vi "Modify VI Settings.vi"() -> ()   [LabVIEW 2013]
uses:
  ReentrancyType--Enum.ctl
panel:
  in  "Set Reentrancy Type":bool=TRUE
  in  "Set Inline":bool=TRUE
  in  "Set Auto Error Handling":bool=TRUE
  in  "Set Debugging":bool=TRUE
  in  "Path":path=path "C:/Project/JKI-Internal/OpenG-Variant-Data-Library/source"
  in  "Exceptions (VI Names)":string[](array[string])=["Size of Data from TD", "Get Default Data from TD"]
  in  "Reentrancy Type":T1=enum."Preallocate Reentrant"
  in  "Inline":bool=TRUE
  in  "Automatic Error Handling":bool
  in  "Debugging":bool
  # "Settings"
  # "Set?"
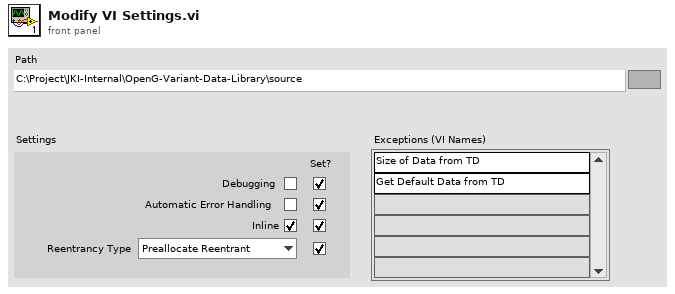
[diagram p1: front panel]
types:
  T1 = typedef "ReentrancyType--Enum.ctl" = enum16{"Non Reentrant", "Shared Clones Reentrant", "Preallocate Reentrant"}
  T2 = enum32{"invalid VI type", "Standard VI", "Control VI", "Global VI", "Polymorphic VI", "Configuration VI", "SubSystem", "Facade VI", "Method VI", "Statechart Diagram VI"}
  T3 = enum16{"Share clones between instances", "Preallocate clone for each instance"}
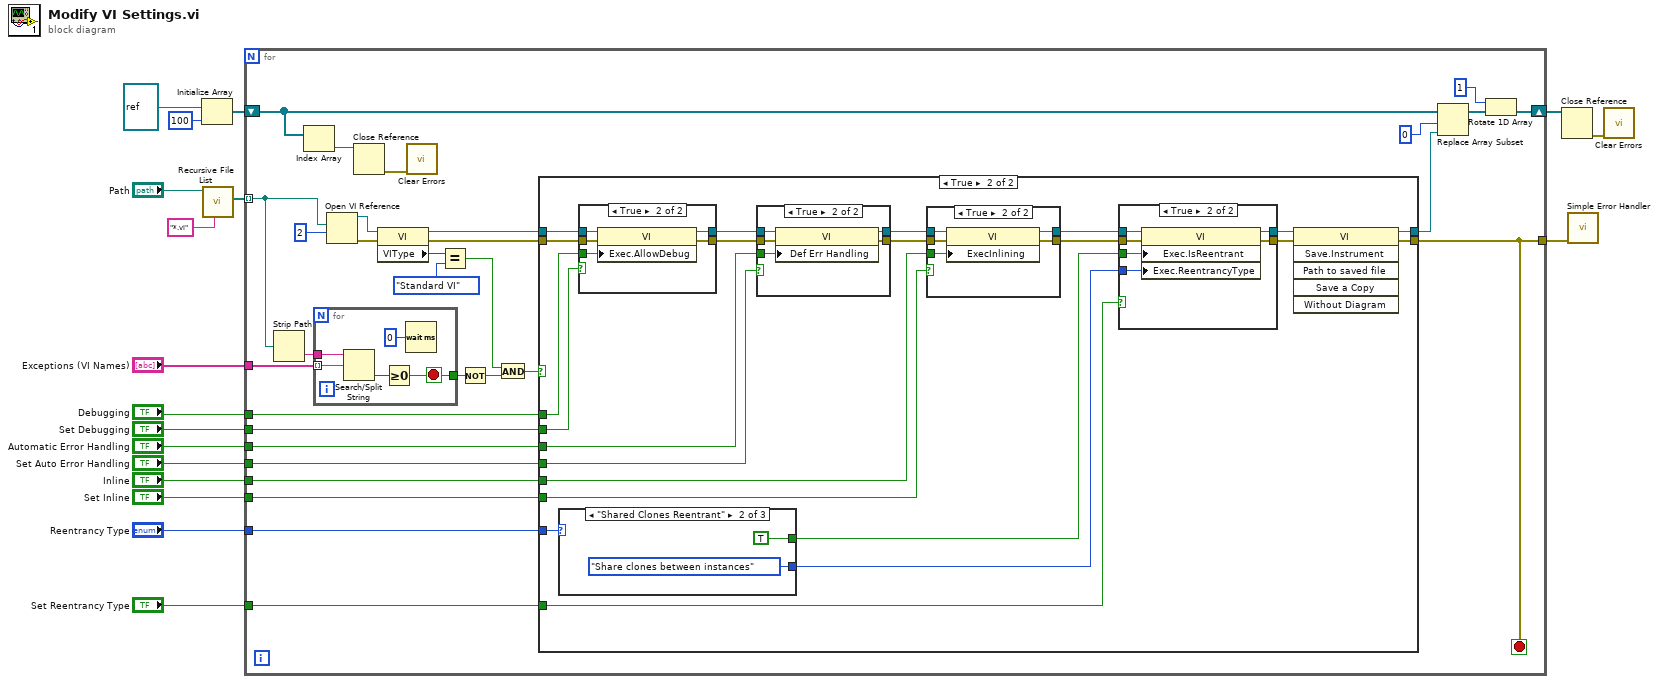
[diagram p0: block diagram]
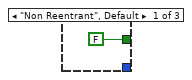
[diagram p7: hidden frame]
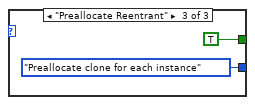
[diagram p8: hidden frame]
diagram:
  n1 = Initialize Array(refnum<vi> refnum ("vi reference"), 100 ("dimension size")) -> (w15:refnum<vi>[])
  n2 = call <vilib>:"Recursive File List.vi"("pattern"="*.vi", "Folder Path"="Path") -> ("All Files in Dir"=w13:path[])  [unwired: 5 in, 4 out]
  n3 = for {
    tunnel: w13 -> [w46] mode=indexing
    tunnel: "Debugging" -> [w48]
    tunnel: "Automatic Error Handling" -> [w47]
    tunnel: "Exceptions (VI Names)" -> [w45]
    shift-right: [w41] -> w7
    shift-left: w15 -> [w39]
    tunnel: [w30] -> w14
    tunnel: "Reentrancy Type" -> [w32]
    tunnel: "Inline" -> [w31]
    tunnel: "Set Debugging" -> [w22]
    tunnel: "Set Auto Error Handling" -> [w21]
    tunnel: "Set Inline" -> [w20]
    tunnel: "Set Reentrancy Type" -> [w19]
    stop <- w30 stop-if-true
    n4 = Strip Path(path=w46) -> (name=w44:string)  [unwired: 1 out]
    n5 = Index Array(array=w39) -> (element=w38:refnum<vi>)  [unwired: 1 in]
    n6 = for {
      tunnel: w45 -> [w110] mode=indexing
      tunnel: w44 -> [w111]
      tunnel: [w108] -> w26
      stop <- w108 stop-if-true
      n7 = Search/Split String(string=w111, search string/char (-)=w110) -> (offset of match=w112:i32)  [unwired: 1 in, 2 out]
      n8 = Greater Or Equal To 0?(x=w112) -> (x >= 0?=w108:bool)
      n9 = Wait (ms)(milliseconds to wait=u32 0) -> ()  [unwired: 1 out]
    }
    n10 = Open VI Reference(vi path=w46, options=2) -> (vi reference=w34:refnum<vi>, error out=w49:errorcluster)  [unwired: 4 in]
    n11 = Close Reference(reference=w38) -> (error out=w37:errorcluster)  [unwired: 1 in]
    n12 = property class="VI"(reference=w34, error in=w49) -> (reference out=w33:refnum<vi>, error out=w35:errorcluster, "VIType"=w28:T2)
    n13 = call <vilib>:"Clear Errors.vi"("error in (no error)"=w37) -> ()  [unwired: 6 in, 1 out]
    n14 = Equal?(x=w28, y=T2."Standard VI") -> (x = y?=w27:bool)
    n15 = Not(x=w26) -> (.not. x?=w25:bool)
    n16 = And(x=w27, y=w25) -> (x .and. y?=w24:bool)
    n17 = case shown="True" w24 {
      tunnel: w48 -> [_ w64]
      tunnel: w47 -> [_ w60]
      tunnel: [w50 w71] -> w29
      tunnel: [w51 w70] -> w30
      tunnel: w35 -> [w51 w65]
      tunnel: w33 -> [w50 w66]
      tunnel: w32 -> [_ w67]
      tunnel: w31 -> [_ w55]
      tunnel: w22 -> [_ w63]
      tunnel: w21 -> [_ w59]
      tunnel: w20 -> [_ w54]
      tunnel: w19 -> [_ w52]
      frame False {
      }
      frame True {
        n18 = case shown="\"Shared Clones Reentrant\"" w67 {
          tunnel: [_ T3."Share clones between instances" ("Execution:Reentrancy Type") T3."Preallocate clone for each instance" ("Execution:Reentrancy Type")] -> w69
          tunnel: [FALSE TRUE TRUE] -> w68
          frame "Non Reentrant", Default {
          }
          frame "Shared Clones Reentrant" {
          }
          frame "Preallocate Reentrant" {
          }
        }
        n19 = case shown="True" w63 {
          tunnel: w66 -> [w97 w102]
          tunnel: [w97 w101] -> w62
          tunnel: w65 -> [w96 w100]
          tunnel: [w96 w99] -> w61
          tunnel: w64 -> [_ w98]
          frame False {
          }
          frame True {
            n20 = property class="VI"(reference=w102, error in=w100, "Exec.AllowDebug"=w98) -> (reference out=w101:refnum<vi>, error out=w99:errorcluster)
          }
        }
        n21 = case shown="True" w59 {
          tunnel: w62 -> [w90 w95]
          tunnel: [w90 w94] -> w57
          tunnel: [w89 w93] -> w58
          tunnel: w61 -> [w89 w92]
          tunnel: w60 -> [_ w91]
          frame False {
          }
          frame True {
            n22 = property class="VI"(reference=w95, error in=w92, "Def Err Handling"=w91) -> (reference out=w94:refnum<vi>, error out=w93:errorcluster)
          }
        }
        n23 = case shown="True" w54 {
          tunnel: w58 -> [w82 w88]
          tunnel: w57 -> [w83 w87]
          tunnel: [w83 w86] -> w56
          tunnel: w55 -> [_ w85]
          tunnel: [w82 w84] -> w53
          frame False {
          }
          frame True {
            n24 = property class="VI"(reference=w87, error in=w88, "ExecInlining"=w85) -> (reference out=w86:refnum<vi>, error out=w84:errorcluster)
          }
        }
        n25 = case shown="True" w52 {
          tunnel: [w74 w81] -> w73
          tunnel: [w75 w80] -> w72
          tunnel: w69 -> [_ w79]
          tunnel: w68 -> [_ w78]
          tunnel: w56 -> [w75 w77]
          tunnel: w53 -> [w74 w76]
          frame False {
          }
          frame True {
            n26 = property class="VI"(reference=w77, error in=w76, "Exec.IsReentrant"=w78, "Exec.ReentrancyType"=w79) -> (reference out=w80:refnum<vi>, error out=w81:errorcluster)
          }
        }
        n27 = invoke class="VI" method="Save.Instrument"(reference=w72, error in=w73) -> (reference out=w71:refnum<vi>, error out=w70:errorcluster)  [unwired: 4 in, 4 out]
      }
    }
    n28 = Replace Array Subset(array=w39, new element=w29, index=0) -> (w43:refnum<vi>[])
    n29 = Rotate 1D Array(1:w43, 2:1 ("n")) -> (0:w41:refnum<vi>[])
  }
  n30 = Close Reference(reference=w7) -> (error out=w6:errorcluster)  [unwired: 1 in]
  n31 = call <vilib>:"Simple Error Handler.vi"("error in (no error)"=w14) -> ()  [unwired: 4 in, 5 out]
  n32 = call <vilib>:"Clear Errors.vi"("error in (no error)"=w6) -> ()  [unwired: 6 in, 1 out]
